vi "interval_move.vi"(5 "Interval (s)":dbl=0.1, 7 "Speed(um/s)":dbl=1.0, 8 "error in":errorcluster, 9 "handle":i32, 10 "axis":i32, 11 "Destination":dbl) -> (0 "error out":errorcluster, 1 "handle out":i32, 2 "axis out":i32, 3 "position":dbl)   [LabVIEW 2026]
uses:
  Madlib.dll
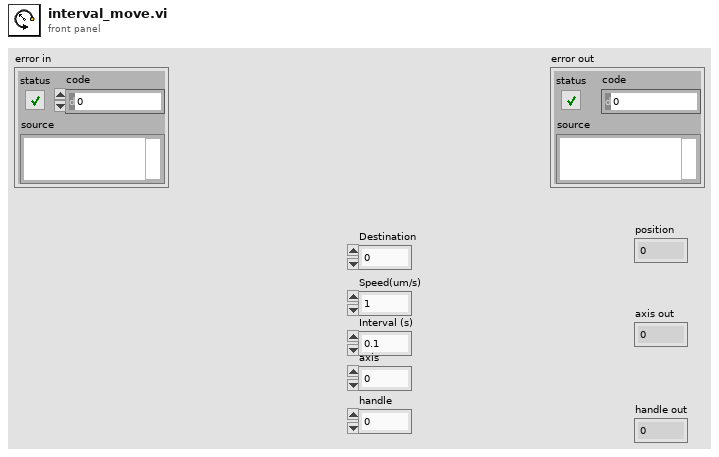
[diagram p1: front panel]
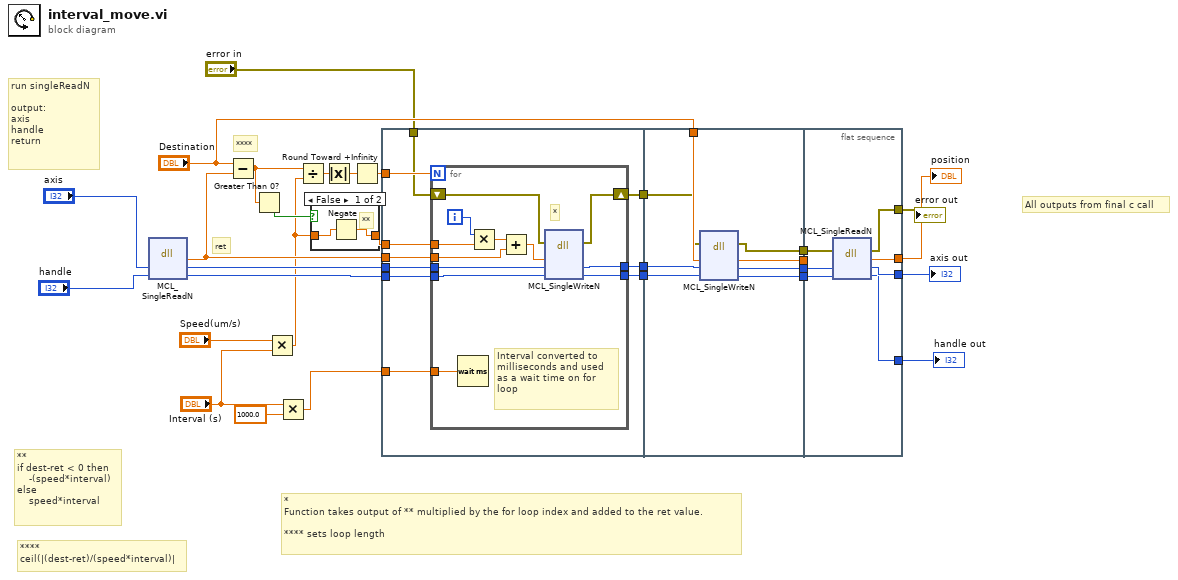
[diagram p0: block diagram]
diagram:
  # "All outputs from final c call"
  # "*\nFunction takes output of ** multiplied by the for loop index and added to the ret value.\n\n**** sets loop length"
  # "**\nif dest-ret < 0 then \n    -(speed*interval) \nelse \n    speed*interval"
  # "****\nceil(|(dest-ret)/(speed*interval)|"
  # "****"
  # "ret"
  # "run singleReadN\n\noutput:\naxis\nhandle\nreturn"
  n1 = dll-call lib="\\\\userfs\\psmr500/w2k/Desktop/COMBI-Tweez/COMBI-Tweez-main/LabVIEW Microscope Control/Nanostage/Madlib.dll" fn="MCL_SingleReadN"("axis"="axis", "handle"="handle") -> ("return type"=w24:dbl, "axis"=w19:i32, "handle"=w20:i32)  [unwired: 3 in, 2 out]
  n2 = Subtract(x="Destination", y=w24) -> (x-y=w15:dbl)
  n3 = Greater Than 0?(x=w15) -> (x > 0?=w14:bool)
  n4 = Multiply(x="Speed(um/s)", y="Interval (s)") -> (x*y=w12:dbl)
  n5 = Multiply(x="Interval (s)", y=1000.0) -> (x*y=w25:dbl)
  n6 = Divide(x=w15, y=w12) -> (x/y=w18:dbl)
  n7 = case shown="False" w14 {
    tunnel: w12 -> [w30 w32]
    tunnel: [w31 w32] -> w13
    frame False {
      # "**"
      n8 = Negate(x=w30) -> (-x=w31:dbl)
    }
    frame True {
    }
  }
  n9 = Absolute Value(x=w18) -> (abs(x)=w16:dbl)
  n10 = Round Toward +Infinity(x=w16) -> (ceil(x): smallest int >= x=w17:dbl)
  n11 = flat-sequence {
    tunnel: w17 -> [w42]
    tunnel: w25 -> [w41]
    tunnel: w13 -> [w40]
    tunnel: w24 -> [w39]
    tunnel: [w38] -> w23
    tunnel: [w37] -> w22
    tunnel: w20 -> [w36]
    tunnel: w19 -> [w35]
    tunnel: [w34] -> w4
    tunnel: "error in" -> [w33]
    tunnel: w23 -> [w62]
    tunnel: w22 -> [w61]
    tunnel: "Destination" -> [w60]
    tunnel: [w59] -> w11
    tunnel: [w58] -> w10
    tunnel: [w57] -> w9
    tunnel: w4 -> [w56]
    tunnel: [w55] -> w3
    tunnel: w11 -> [w68]
    tunnel: w10 -> [w69]
    tunnel: w9 -> [_]
    tunnel: [w66] -> w8
    tunnel: [w67] -> w7
    tunnel: [w65] -> w5
    tunnel: w3 -> [w64]
    tunnel: [w63] -> w2
    frame #0 {
      n12 = for {
        N: w42 -> [_]
        tunnel: w41 -> [w54]
        tunnel: w40 -> [w53]
        tunnel: w39 -> [w51]
        tunnel: [w49] -> w38
        tunnel: [w48] -> w37
        tunnel: w36 -> [w47]
        tunnel: w35 -> [w46]
        shift-right: [w43] -> w34
        shift-left: w33 -> [w44]
        i -> [w45]
        # "*"
        # "Interval converted to \nmilliseconds and used \nas a wait time on for\nloop"
        n13 = Wait (ms)(milliseconds to wait=w54) -> ()  [unwired: 1 out]
        n14 = Multiply(x=w45, y=w53) -> (x*y=w52:dbl)
        n15 = Add(x=w52, y=w51) -> (x+y=w50:dbl)
        n16 = dll-call lib="\\\\userfs\\psmr500/w2k/Desktop/COMBI-Tweez/COMBI-Tweez-main/LabVIEW Microscope Control/Nanostage/Madlib.dll" fn="MCL_SingleWriteN"(error in=w44, "position"=w50, "axis"=w46, "handle"=w47) -> (error out=w43:errorcluster, "axis"=w48:i32, "handle"=w49:i32)  [unwired: 4 in, 1 out]
      }
    }
    frame #1 {
      n17 = dll-call lib="\\\\userfs\\psmr500/w2k/Desktop/COMBI-Tweez/COMBI-Tweez-main/LabVIEW Microscope Control/Nanostage/Madlib.dll" fn="MCL_SingleWriteN"(error in=w56, "position"=w60, "axis"=w61, "handle"=w62) -> (error out=w55:errorcluster, "position"=w57:dbl, "axis"=w59:i32, "handle"=w58:i32)  [unwired: 3 in, 1 out]
    }
    frame #2 {
      n18 = dll-call lib="\\\\userfs\\psmr500/w2k/Desktop/COMBI-Tweez/COMBI-Tweez-main/LabVIEW Microscope Control/Nanostage/Madlib.dll" fn="MCL_SingleReadN"(error in=w64, "axis"=w68, "handle"=w69) -> (error out=w63:errorcluster, "return type"=w66:dbl, "axis"=w67:i32, "handle"=w65:i32)  [unwired: 2 in, 1 out]
    }
  }
  "position" <- w8
  "axis out" <- w7
  "handle out" <- w5
  "error out" <- w2
